vi "Get Current Skin.vi"(4 "default":picture, 5 "error in (no error)":errorcluster, 8 "Object":string) -> (0 "error out":errorcluster, 1 "image data":T1, 2 "Picture with skin":picture)   [LabVIEW 2026, in "TALOS.lvlib"]
uses:
  TALOS.lvlib
  <vilib>/picture/picture.llb/imagedata.ctl
  Ancestor/Ancestor/Ancestor.lvclass/Ancestor.ctl
  Generate Error.vi
  FGV/Error Memory/Get Error Description.vi
  Get PC name.vi
  Ancestor/Ancestor/Read ID.vi
  Get Class Name.vi
  <vilib>/Utility/error.llb/Clear Errors.vi
  FGV/Error Memory/Error Memory Core.vi
  <vilib>/AdvancedString/Delimited String to 1D String Array.vi
  <vilib>/AdvancedString/Delimited String to 1D String Array (string).vi
  FGV/Error Memory/Error Crt Lvl checker.vi
  FGV/Error Memory/Error Memory Core.vi/40c8088d-b597-4017-91af-faa98e00292e.vi
  FGV/Error Memory/Error Memory Core.vi/d4a3ab98-063c-4e44-b43d-fbdcfe6c2be2.vi
  Global Memory.vi
  <vilib>/Utility/LVClass/Get LV Class Name.vi
  Is in Packed Library.vi
  TALOS Root path.vi
  Read CSV worksheet.vi
  Global Constants.vi
  <vilib>/Utility/error.llb/General Error Handler.vi
  <vilib>/Utility/config.llb/Open Config Data.vi
  <vilib>/Utility/config.llb/Get Section Names.vi
  <vilib>/Utility/config.llb/Get Key Names.vi
  <vilib>/Utility/config.llb/Read Key.vi
  <vilib>/Utility/config.llb/Read Key (String).vi
  <vilib>/Utility/config.llb/Close Config Data.vi
  Ancestor/Ancestor/Ancestor.lvclass
  <vilib>/Comparison/Equal/Equal Functor/Equal Functor.lvclass
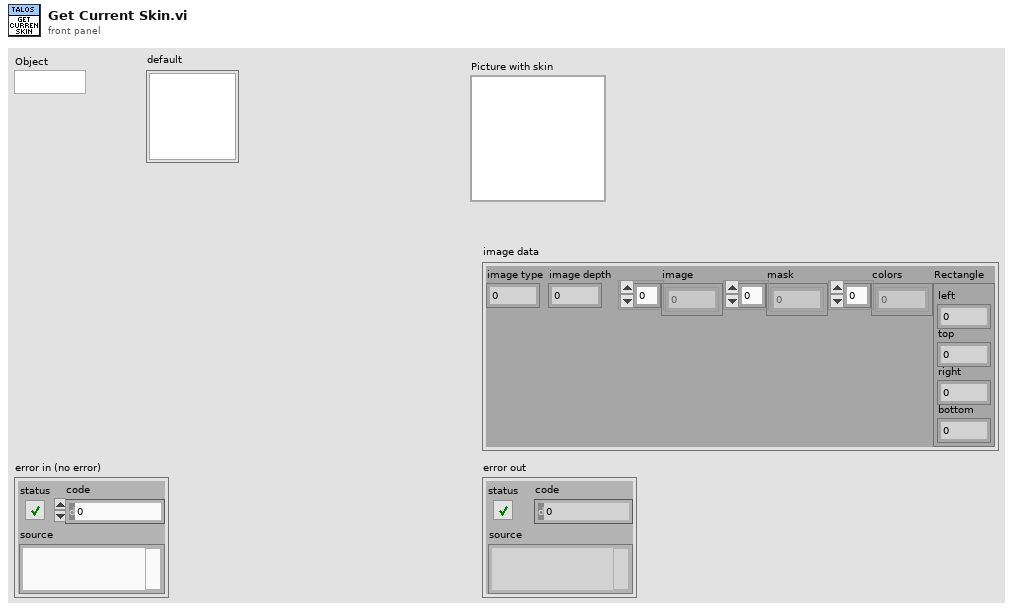
[diagram p1: front panel]
types:
  T1 = typedef "imagedata.ctl" = cluster{"image type":i32, "image depth":i32, "image":u8[], "mask":u8[], "colors":u32[], "Rectangle":cluster{"left":i16, "top":i16, "right":i16, "bottom":i16}}
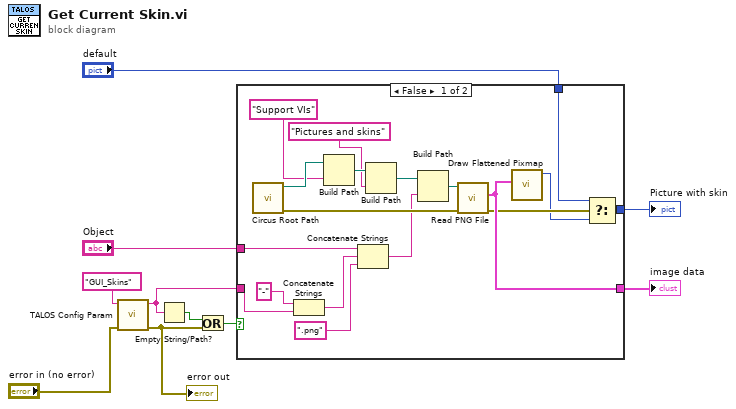
[diagram p0: block diagram]
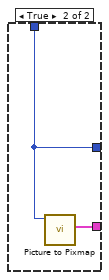
[diagram p2: hidden frame]
diagram:
  n1 = call "TALOS Config Param.vi"("error in (no error)"="error in (no error)", "Parameter Name"="GUI_Skins") -> ("error out"=w6:errorcluster, "Output"=w4:string)  [unwired: 8 in]
  "error out" <- w6
  n2 = Empty String/Path?(string/path=w4) -> (empty?=w5:bool)
  n3 = Or(x=w5, y=w6) -> (x .or. y?=w2:bool)
  n4 = case shown="False" w2 {
    tunnel: "Object" -> [w21 _]
    tunnel: [w19 w29] -> w9
    tunnel: [w18 w30] -> w8
    tunnel: w4 -> [w15 _]
    tunnel: "default" -> [w12 w30]
    frame False {
      n5 = call "Circus Root Path.vi"() -> ("error out"=w26:errorcluster, "Circus Root Path"=w28:path)  [unwired: 10 in]
      n6 = Concatenate Strings("-" ("string"), w15) -> (w16:string)
      n7 = Build Path(base path=w28, name or relative path="Support VIs") -> (appended path=w27:path)
      n8 = Concatenate Strings(w21, w16, ".png" ("string")) -> (w20:string)
      n9 = Build Path(base path=w27, name or relative path="Pictures and skins") -> (appended path=w25:path)
      n10 = Build Path(base path=w25, name or relative path=w20) -> (appended path=w24:path)
      n11 = call <vilib>:"Read PNG File.vi"("error in (no error)"=w26, "path to PNG file"=w24) -> ("error out"=w13:errorcluster, "image data"=w19:T1)  [unwired: 7 in, 1 out]
      n12 = call <vilib>:"Draw Flattened Pixmap.vi"("image data"=w19) -> ("new picture"=w11:picture)  [unwired: 8 in]
      n13 = Select(t=w12, s=w13, f=w11) -> (s? t:f=w18:picture)
    }
    frame True {
      n14 = call <vilib>:"Picture to Pixmap.vi"("picture"=w30) -> ("image data"=w29:T1)  [unwired: 9 in, 1 out]
    }
  }
  "Picture with skin" <- w8
  "image data" <- w9
